vi "灭火装置参数配置.vi"() -> ()   [LabVIEW 2016, in "环境动力监测库.lvlib"]
panel:
  in  "启用烟雾监测":bool
  in  "功能启用":bool
  in  "开启温度":dbl=60.0 format="%#.2f ℃"
  # "灭火装置参数配置"
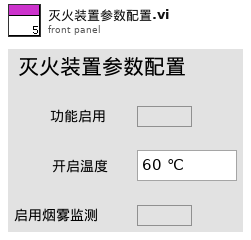
[diagram p1: front panel]
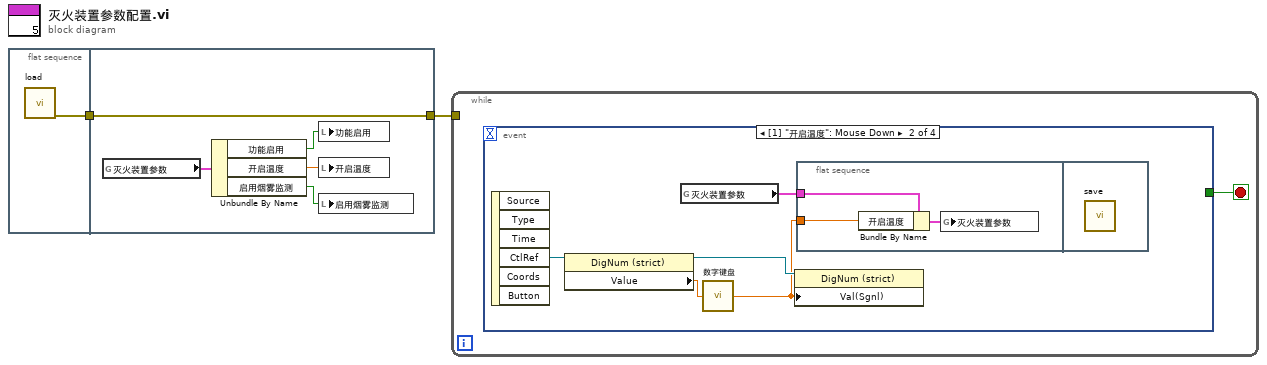
[diagram p0: block diagram]
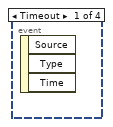
[diagram p2: hidden frame]
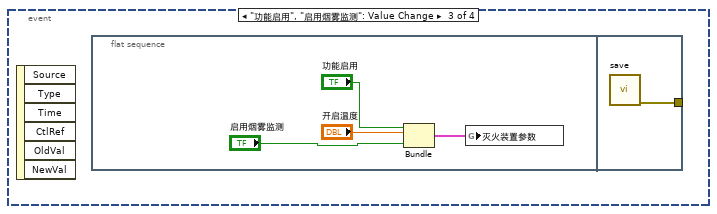
[diagram p3: hidden frame]
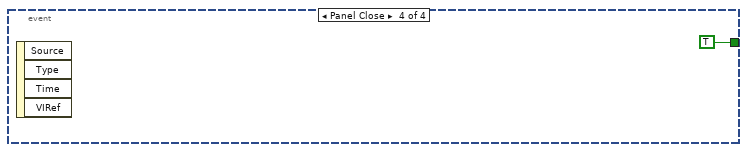
[diagram p4: hidden frame]
diagram:
  n1 = flat-sequence {
    tunnel: [w3] -> w2
    tunnel: [w8] -> w1
    tunnel: w2 -> [w8]
    frame #0 {
      n2 = call "load.vi"() -> ("error out"=w3:errorcluster)  [unwired: 11 in]
    }
    frame #1 {
      n3 = global read "断电保存全局变量.vi" "灭火装置参数"() -> (w7:cluster{"功能启用":bool, "开启温度":dbl, "启用烟雾监测":bool})
      n4 = Unbundle By Name(w7) -> ("功能启用"=w6:bool, "开启温度"=w5:dbl, "启用烟雾监测"=w4:bool)
      n5 = local write "功能启用"(w6) -> ()
      n6 = local write "开启温度"(w5) -> ()
      n7 = local write "启用烟雾监测"(w4) -> ()
    }
  }
  n8 = while {
    tunnel: w1 -> [_]
    stop <- w9 stop-if-true
    n9 = event shown="[1] \"开启温度\": Mouse Down" {
      selector: _ -> [_ _ _ _]
      dyn-events: _ -> [_ _ _ _]
      timeout: _ -> [_ _ _ _]
      tunnel: [_ _ _ TRUE] -> w9
      event Timeout {
        n10 = event-data() -> ()  [unwired: 1 in, 3 out]
      }
      event "开启温度": Mouse Down {
        n11 = event-data() -> ("CtlRef"=w14:refnum<vi>)  [unwired: 1 in, 5 out]
        n12 = property class="DigNum (strict)"(reference=w14) -> (reference out=w12:refnum<vi>, "Value"=w13:dbl)  [unwired: 1 in, 1 out]
        n13 = global read "断电保存全局变量.vi" "灭火装置参数"() -> (w11:cluster{"功能启用":bool, "开启温度":dbl, "启用烟雾监测":bool})
        n14 = call "数字键盘.vi"("OldNumber"=w13) -> ("NewNumber"=w10:sgl)
        n15 = property class="DigNum (strict)"(reference=w12, "Val(Sgnl)"=w10) -> ()  [unwired: 1 in, 2 out]
        n16 = flat-sequence {
          tunnel: w11 -> [w17]
          tunnel: w10 -> [w16]
          frame #0 {
            n17 = Bundle By Name(cluster=w17, "开启温度"=w16) -> (w15:cluster{"功能启用":bool, "开启温度":dbl, "启用烟雾监测":bool})
            n18 = global write "断电保存全局变量.vi" "灭火装置参数"(w15) -> ()
          }
          frame #1 {
            n19 = call "save.vi"() -> ()  [unwired: 11 in, 1 out]
          }
        }
      }
      event "功能启用", "启用烟雾监测": Value Change {
        n20 = event-data() -> ()  [unwired: 1 in, 6 out]
        n21 = flat-sequence {
          tunnel: [w22] -> _
          frame #0 {
            n22 = Bundle("功能启用"="功能启用", "开启温度"="开启温度", "启用烟雾监测"="启用烟雾监测") -> (w21:cluster{"功能启用":bool, "开启温度":dbl, "启用烟雾监测":bool})  [unwired: 1 in]
            n23 = global write "断电保存全局变量.vi" "灭火装置参数"(w21) -> ()
          }
          frame #1 {
            n24 = call "save.vi"() -> ("error out"=w22:errorcluster)  [unwired: 11 in]
          }
        }
      }
      event Panel Close {
        n25 = event-data() -> ()  [unwired: 1 in, 4 out]
      }
    }
  }
